vi "Fact.vi"() -> ()   [LabVIEW 2019, in "LVUnitTestBuilderTest.lvlib" / "LibraryWithFact.lvlib"]
uses:
  LibraryWithFact.lvlib
panel:
  out "error out":errorcluster
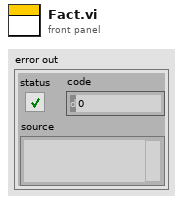
[diagram p1: front panel]
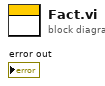
[diagram p0: block diagram]
diagram:
